vi "WaveAverager.vi"(8 "Reset":bool, 11 "waveform":waveform(dbl)) -> (3 "output waveform":waveform(dbl))   [LabVIEW 2014]
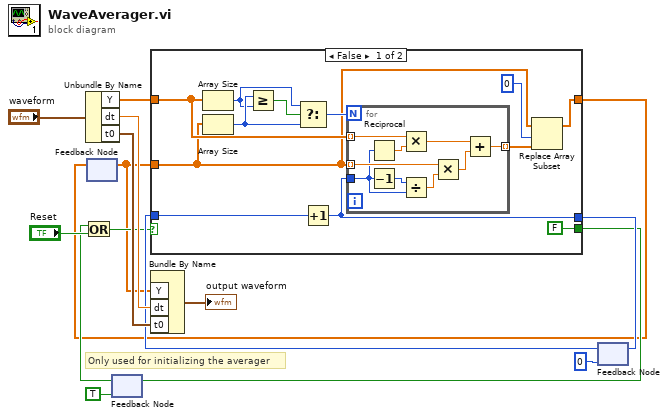
[diagram p0: block diagram]
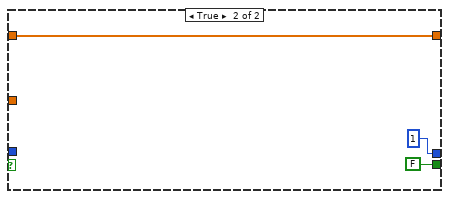
[diagram p2: hidden frame]
diagram:
  # "Only used for initializing the averager"
  n1 = Unbundle By Name("waveform") -> ("Y"=w15:dbl[], "dt"=w13:dbl, "t0"=w12:timestamp)
  n2 = feedback #1() -> (w2:dbl[])  [unwired: 1 in]
  n3 = feedback #2(TRUE) -> (w5:bool)
  n4 = Or(x=w5, y="Reset") -> (x .or. y?=w7:bool)
  n5 = Bundle By Name("Y"=w2, "dt"=w13, "t0"=w12) -> (→"output waveform":waveform(dbl))  [unwired: 1 in]
  n6 = feedback #3(0) -> (w9:i32)
  n7 = case shown="False" w7 {
    tunnel: w15 -> [w21 w39]
    tunnel: [w19 w39] -> w3
    tunnel: [w20 1] -> w11
    tunnel: w9 -> [w27 _]
    tunnel: [FALSE FALSE] -> w6
    tunnel: w2 -> [w18 _]
    frame False {
      n8 = Array Size(array=w21) -> (size(s)=w23:i32)
      n9 = Array Size(array=w18) -> (size(s)=w24:i32)
      n10 = Greater Or Equal?(x=w24, y=w23) -> (x >= y?=w25:bool)
      n11 = Select(t=w23, s=w25, f=w24) -> (s? t:f=w22:i32)
      n12 = Increment(x=w27) -> (x+1=w20:i32)
      n13 = for {
        N: w22 -> [_]
        tunnel: w21 -> [w36] mode=indexing
        tunnel: w20 -> [w32]
        tunnel: w18 -> [w34] mode=indexing
        tunnel: [w28] -> w16 mode=indexing
        n14 = Reciprocal(x=w32) -> (1/x=w35:dbl)
        n15 = Decrement(x=w32) -> (x-1=w33:i32)
        n16 = Multiply(x=w36, y=w35) -> (x*y=w29:dbl)
        n17 = Divide(x=w33, y=w32) -> (x/y=w31:dbl)
        n18 = Multiply(x=w34, y=w31) -> (x*y=w30:dbl)
        n19 = Add(x=w29, y=w30) -> (x+y=w28:dbl)
      }
      n20 = Replace Array Subset(array=w18, new element=w16, index=0) -> (w19:dbl[])
    }
    frame True {
    }
  }
  n21 = feedback-in #1(w3) -> ()
  n22 = feedback-in #2(w6) -> ()
  n23 = feedback-in #3(w11) -> ()
